vi "file list from temperatures file V3.vi"(6 "monotonic segments ON/OFF":bool=TRUE, 7 "action":T4(ring)=enum."update monotonic pieces", 9 "tfolder IN":T1={"tfolder path"=path "/snowfall/Users/arcadi/Desktop/Ultrasound/Experiment/YBCO_4/Round1/Sweep12/June_2011/062511/221.16400K_300_3100_001_062511.dat", "9folder path"=path "/snowfall/Users/arcadi/Desktop/Ultrasound/Experiment/YBCO_4/Round1/Sweep12/June_2011/062511/221.16400K_300_3100_001_062511.dat", "tfolder  -  file array"=[], "from index array"=[], "timestamp array"=[]}, 11 "tfolder file path  IN":path=path "/snowfall/Users/arcadi/Desktop/Ultrasound/Experiment/YBCO_4/Round1/Sweep12/June_2011/062511/221.16400K_300_3100_001_062511.dat") -> (0 "timestamp OUT":dbl[](array[numeric]), 1 "tfolder OUT":T1={"tfolder path"=path "/snowfall/Users/arcadi/Desktop/Ultrasound/Experiment/YBCO_4/Round1/Sweep12/June_2011/062511/221.16400K_300_3100_001_062511.dat", "9folder path"=path "/snowfall/Users/arcadi/Desktop/Ultrasound/Experiment/YBCO_4/Round1/Sweep12/June_2011/062511/221.16400K_300_3100_001_062511.dat", "tfolder  -  file array"=[], "from index array"=[], "timestamp array"=[]}, 2 "sweep path array OUT":T3[](array[typedef]), 3 "temperature OUT":dbl[](array[numeric]), 5 "OK":bool)   [LabVIEW 2010]
uses:
  sweep file name.ctl
  tfolder -- monotonic segment.ctl
  tfolder.ctl
panel:
  in  "tfolder - monotonic segment":T2
  in  "sweep file name":T3={"temperature"=0.0, "temperature str"="", "file path"=path "/snowfall/Users/arcadi/Desktop/Ultrasound/Experiment/YBCO_4/Round1/Sweep12/June_2011/062511/221.16400K_300_3100_001_062511.dat", "last mod"=timestamp(0 s since 1904-01-01), "file name str"="", "mod time(min)"=0.0, "file format"=enum.""}
  in  "file path OK":bool=TRUE
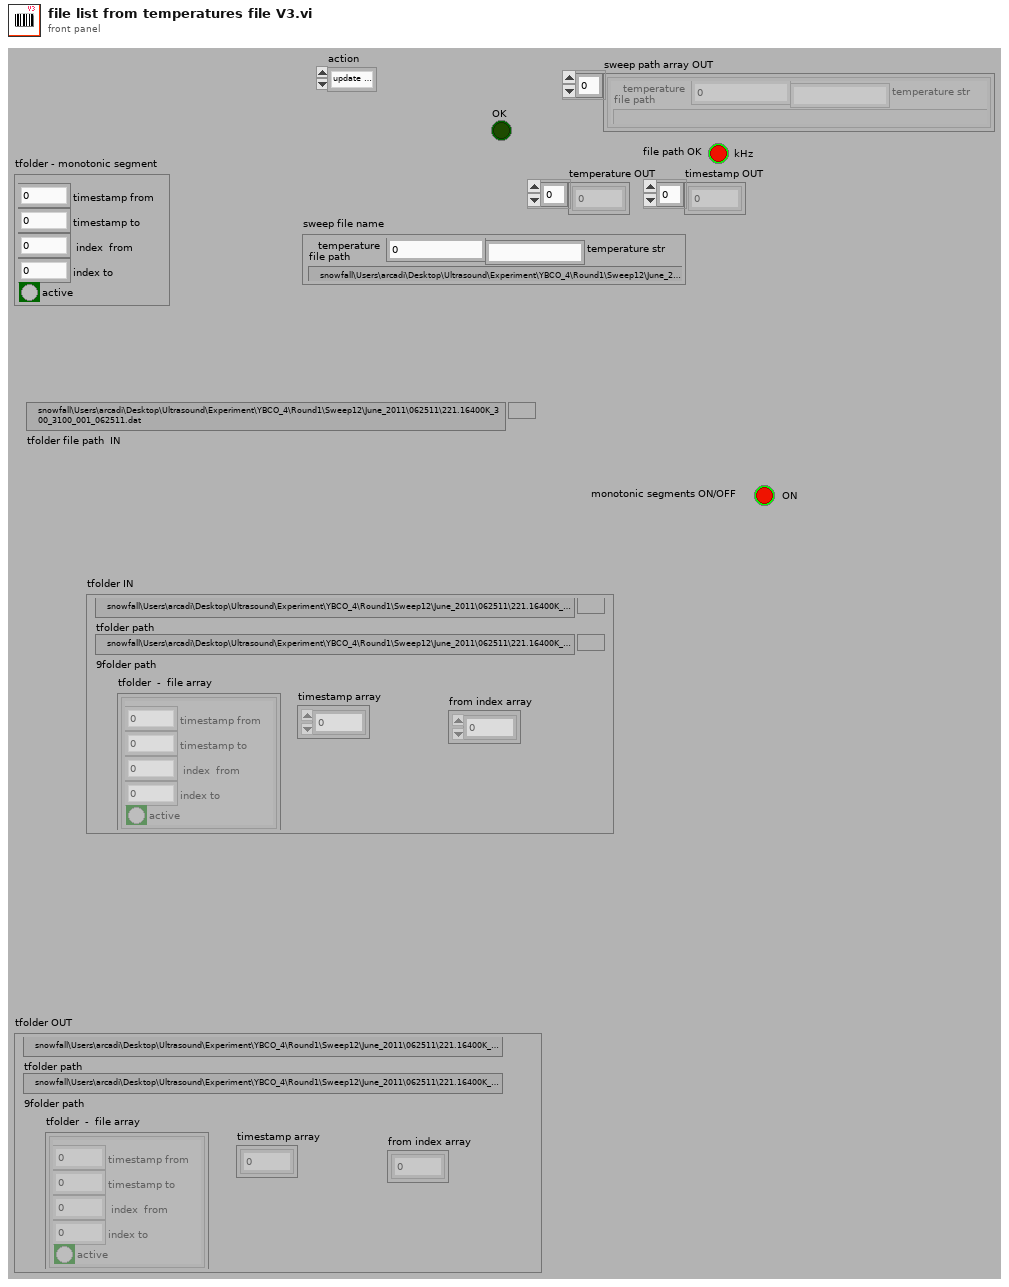
[diagram p1: front panel]
types:
  T1 = typedef "tfolder.ctl" = cluster{"tfolder path":path, "9folder path":path, "tfolder  -  file array":T2[], "from index array":i32[], "timestamp array":dbl[]}
  T2 = typedef "tfolder -- monotonic segment.ctl" = cluster{"timestamp from":dbl, "timestamp to":dbl, " index  from":i32, "index to":i32, "active":bool}
  T3 = typedef "sweep file name.ctl" = cluster{"temperature":dbl, "temperature str":string, "file path":path, "last mod":timestamp, "file name str":string, "mod time(min)":dbl, "file format":enum16{"", "ascii", "binary"}}
  T4 = enum16{"new", "update range", "update monotonic pieces", "init", "check", "reset", ""}
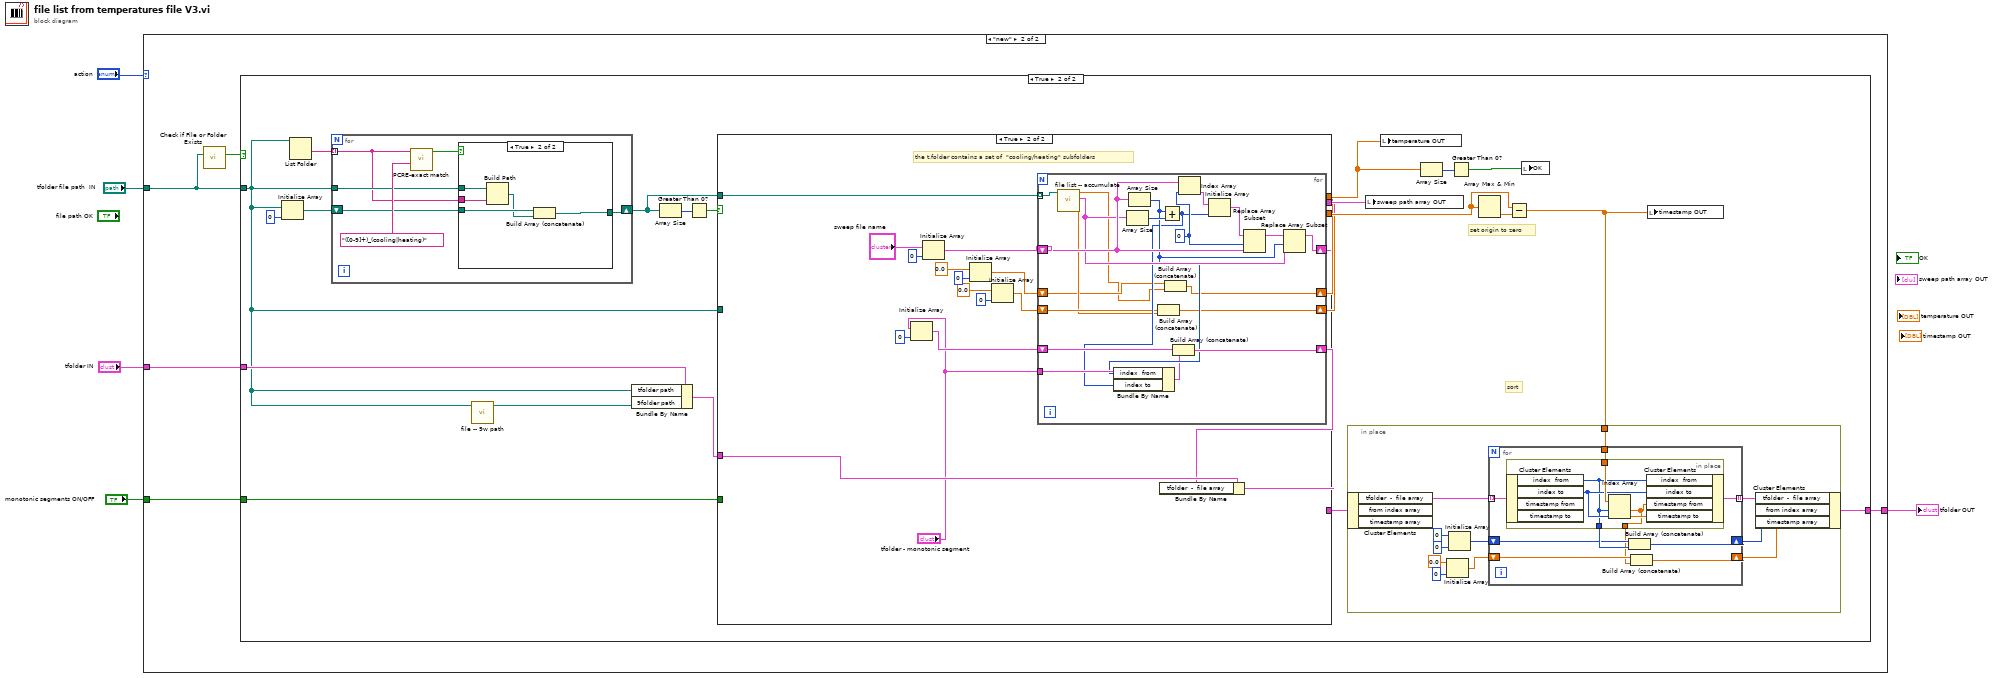
[diagram p0: block diagram]
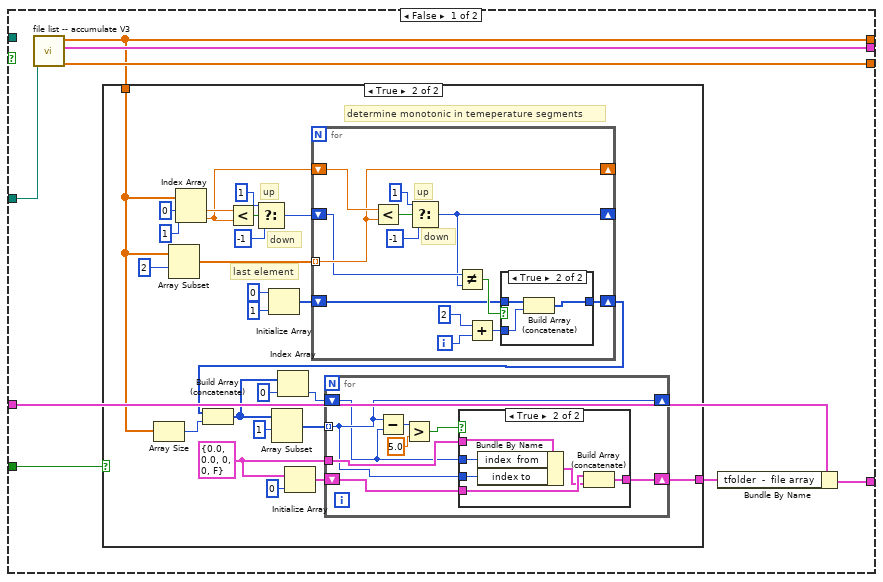
[diagram p4: hidden frame]
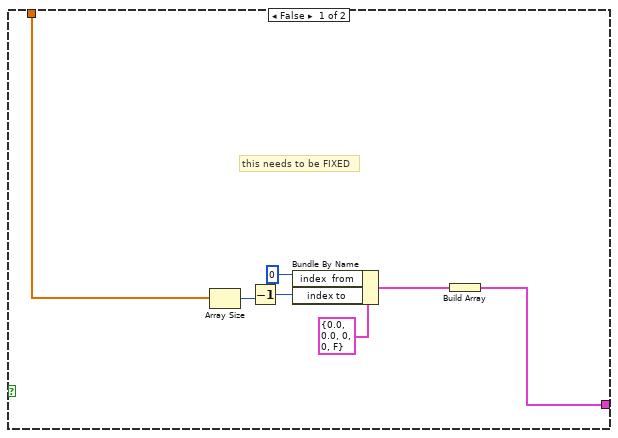
[diagram p5: hidden frame]
diagram:
  n1 = case shown="\"new\"" "action" {
    tunnel: "tfolder file path  IN" -> [_ w10]
    tunnel: "tfolder IN" -> [w6 w9]
    tunnel: [w6 w8] -> w2
    tunnel: "monotonic segments ON/OFF" -> [_ w7]
    frame "", Default {
    }
    frame "new" {
      n2 = call <vilib>:"Check if File or Folder Exists.vi"("path"=w10) -> ("file or folder exists?"=w11:bool)  [unwired: 8 in, 2 out]
      n3 = case shown="True" w11 {
        tunnel: w10 -> [_ w14]
        tunnel: w9 -> [w12 w26]
        tunnel: [w12 w20] -> w8
        tunnel: w7 -> [_ w18]
        frame False {
        }
        frame True {
          # "sort"
          # "set origin to zero"
          n4 = Initialize Array(w14, 0 ("dimension size")) -> (w30:path[])
          n5 = List Folder(path=w14) -> (folder names=w31:string[])  [unwired: 3 in, 3 out]
          n6 = for {
            tunnel: w31 -> [w172] mode=indexing
            shift-right: [w170] -> w27
            shift-left: w30 -> [w171]
            tunnel: w14 -> [w173]
            n7 = call "PCRE-exact match.vi"("regular expression"="([0-9]+)_(cooling|heating)", "input string"=w172) -> ("exact match"=w174:bool)  [unwired: 8 in, 1 out]
            n8 = case shown="True" w174 {
              tunnel: w173 -> [_ w181]
              tunnel: w172 -> [_ w180]
              tunnel: w171 -> [w176 w179]
              tunnel: [w176 w177] -> w170
              frame False {
              }
              frame True {
                n9 = Build Path(base path=w181, name or relative path=w180) -> (appended path=w178:path)
                n10 = Build Array (concatenate)(w179, w178) -> (w177:path[])
              }
            }
          }
          n11 = call "file -- 9w path.vi"("sweep folder"=w14) -> ("9w path"=w13:path)  [unwired: 10 in]
          n12 = Bundle By Name(cluster=w26, "tfolder path"=w14, "9folder path"=w13) -> (w24:T1)
          n13 = Array Size(array=w27) -> (size(s)=w29:i32)
          n14 = Greater Than 0?(x=w29) -> (x > 0?=w28:bool)
          n15 = case shown="True" w28 {
            tunnel: w27 -> [_ w148]
            tunnel: [w60 w147] -> w22
            tunnel: [w59 w146] -> w16
            tunnel: [w65 w145] -> w25
            tunnel: w24 -> [w63 w142]
            tunnel: [w62 w141] -> w21
            tunnel: w14 -> [w64 _]
            tunnel: w18 -> [w58 _]
            frame False {
              n16 = call "file list -- accumulate V3.vi"("file path"=w64) -> ("timestamp"=w60:dbl[], "sweep file name array"=w65:T3[], "temperatures"=w59:dbl[])  [unwired: 8 in]
              n17 = case shown="True" w58 {
                tunnel: [w66 w93] -> w61
                tunnel: w59 -> [w71 w73]
                frame False {
                  # "this needs to be FIXED"
                  n18 = Array Size(array=w71) -> (size(s)=w70:i32)
                  n19 = Decrement(x=w70) -> (x-1=w68:i32)
                  n20 = Bundle By Name(cluster=T2 {"timestamp from"=0.0, "timestamp to"=0.0, " index  from"=0, "index to"=0, "active"=FALSE} ("monotonic segment"), "index  from"=0, "index to"=w68) -> (w72:T2)
                  n21 = Build Array(w72) -> (w66:T2[])
                }
                frame True {
                  w94 = T2 {"timestamp from"=0.0, "timestamp to"=0.0, " index  from"=0, "index to"=0, "active"=FALSE} ("monotonic segment")
                  # "determine monotonic in temeperature segments"
                  # "last element"
                  # "down"
                  # "up"
                  n22 = Array Size(array=w73) -> (size(s)=w75:i32)
                  n23 = Array Subset(array=w73, index=2 ("dimension size")) -> (w87:dbl[])  [unwired: 1 in]
                  n24 = Index Array(array=w73, index #1=0 ("dimension size"), index #2=1 ("dimension size")) -> (element #1=w86:dbl, element #2=w85:dbl)
                  n25 = Less?(x=w86, y=w85) -> (x < y?=w77:bool)
                  n26 = Select(t=1 ("dimension size"), s=w77, f=-1 ("dimension size")) -> (s? t:f=w82:i32)
                  n27 = Initialize Array(0 ("dimension size"), 1 ("dimension size")) -> (w92:i32[])
                  n28 = Initialize Array(w94, 0 ("dimension size")) -> (w95:T2[])
                  n29 = for {
                    shift-right: [w98] -> w76
                    shift-left: w92 -> [w100]
                    shift-right: [w106] -> _
                    shift-left: w85 -> [w107]
                    tunnel: w87 -> [w106] mode=indexing
                    shift-right: [w102] -> _
                    shift-left: w82 -> [w103]
                    i -> [w105]
                    # "down"
                    # "up"
                    n30 = Less?(x=w107, y=w106) -> (x < y?=w110:bool)
                    n31 = Select(t=1 ("dimension size"), s=w110, f=-1 ("dimension size")) -> (s? t:f=w102:i32)
                    n32 = Not Equal?(x=w103, y=w102) -> (x != y?=w101:bool)
                    n33 = Add(x=2, y=w105) -> (x+y=w99:i32)
                    n34 = case shown="True" w101 {
                      tunnel: w100 -> [w111 w114]
                      tunnel: w99 -> [_ w113]
                      tunnel: [w111 w112] -> w98
                      frame False {
                      }
                      frame True {
                        n35 = Build Array (concatenate)(w114, w113) -> (w112:i32[])
                      }
                    }
                  }
                  n36 = Build Array (concatenate)(w76, w75) -> (w74:i32[])
                  n37 = Array Subset(array=w74, index=1 ("dimension size")) -> (w78:i32[])  [unwired: 1 in]
                  n38 = Index Array(array=w74, index=0 ("dimension size")) -> (element=w80:i32)
                  n39 = for {
                    shift-right: [w121] -> w93
                    shift-left: w95 -> [w122]
                    tunnel: w94 -> [w120]
                    shift-right: [w117] -> _
                    shift-left: w80 -> [w116]
                    tunnel: w78 -> [w117] mode=indexing
                    n40 = Subtract(x=w117, y=w116) -> (x-y=w119:i32)
                    n41 = Greater?(x=w119, y=5.0) -> (0:w115:bool)
                    n42 = case shown="True" w115 {
                      tunnel: w122 -> [w123 w129]
                      tunnel: [w123 w128] -> w121
                      tunnel: w120 -> [_ w126]
                      tunnel: w117 -> [_ w125]
                      tunnel: w116 -> [_ w124]
                      frame False {
                      }
                      frame True {
                        n43 = Bundle By Name(cluster=w126, "index  from"=w124, "index to"=w125) -> (w127:T2)
                        n44 = Build Array (concatenate)(w129, w127) -> (w128:T2[])
                      }
                    }
                  }
                }
              }
              n45 = Bundle By Name(cluster=w63, "tfolder  -  file array"=w61) -> (w62:T1)
            }
            frame True {
              # "the t.folder contains a set of  \"cooling/heating\" subfolders"
              n46 = Initialize Array("tfolder - monotonic segment", 0 ("dimension size")) -> (w143:T2[])
              n47 = Initialize Array("sweep file name", 0 ("dimension size")) -> (w134:T3[])
              n48 = Initialize Array(0.0 ("dimension size"), 0 ("dimension size")) -> (w133:dbl[])
              n49 = Initialize Array(0.0 ("dimension size"), 0 ("dimension size")) -> (w132:dbl[])
              n50 = for {
                tunnel: w148 -> [w169] mode=indexing
                shift-right: [w161] -> w145
                shift-left: w134 -> [w163]
                shift-right: [w149] -> w146
                shift-left: w133 -> [w151]
                shift-right: [w152] -> w147
                shift-left: w132 -> [w154]
                shift-right: [w159] -> w130
                shift-left: w143 -> [w160]
                tunnel: "tfolder - monotonic segment" -> [w158]
                w165 = 0 ("dimension size")
                n51 = call "file list -- accumulate.vi"("file path"=w169) -> ("timestamp"=w153:dbl[], "sweep file name array"=w162:T3[], "temperatures"=w150:dbl[])  [unwired: 8 in]
                n52 = Array Size(array=w162) -> (size(s)=w168:i32)
                n53 = Array Size(array=w163) -> (size(s)=w157:i32)
                n54 = Build Array (concatenate)(w154, w153) -> (w152:dbl[])
                n55 = Add(x=w157, y=w168) -> (x+y=w156:i32)
                n56 = Bundle By Name(cluster=w158, "index  from"=w157, "index to"=w156) -> (w155:T2)
                n57 = Build Array (concatenate)(w151, w150) -> (w149:dbl[])
                n58 = Build Array (concatenate)(w160, w155) -> (w159:T2[])
                n59 = Index Array(array=w163, index=w165) -> (element=w164:T3)
                n60 = Initialize Array(w164, w156) -> (w167:T3[])
                n61 = Replace Array Subset(array=w167, new element=w163, index=w165) -> (w166:T3[])
                n62 = Replace Array Subset(array=w166, new element=w162, index=w157) -> (w161:T3[])
              }
              n63 = Bundle By Name(cluster=w142, "tfolder  -  file array"=w130) -> (w141:T1)
            }
          }
          n64 = local write "sweep path array OUT"(w25) -> ()
          n65 = local write "temperature OUT"(w16) -> ()
          n66 = Array Size(array=w16) -> (size(s)=w17:i32)
          n67 = Greater Than 0?(x=w17) -> (x > 0?=w15:bool)
          n68 = Array Max & Min(array=w22) -> (min value=w23:dbl)  [unwired: 3 out]
          n69 = Subtract(x=w22, y=w23) -> (x-y=w19:dbl[])
          n70 = in-place {
            in-place-border: w19 -> [w42]
            n71 = in-place-cluster #1(w21) -> ("tfolder  -  file array"=w43:T2[])  [unwired: 2 out]
            n72 = Initialize Array(0.0 ("dimension size"), 0 ("dimension size")) -> (w36:dbl[])
            n73 = Initialize Array(0 ("dimension size"), 0 ("dimension size")) -> (w35:i32[])
            n74 = for {
              tunnel: w43 -> [w52] mode=indexing
              tunnel: w42 -> [w51]
              tunnel: [w50] -> w41 mode=indexing
              shift-right: [w45] -> w33
              shift-left: w35 -> [w47]
              shift-right: [w46] -> w34
              shift-left: w36 -> [w49]
              n75 = in-place {
                in-place-border: w51 -> [w57]
                in-place-border: [w54] -> w48
                in-place-border: [w53] -> w44
                n76 = in-place-cluster #2(w52) -> ("index  from"=w54:i32, "index to"=w55:i32)  [unwired: 2 out]
                n77 = Index Array(array=w57, index #1=w54, index #2=w55) -> (element #1=w53:dbl, element #2=w56:dbl)
                n78 = in-place-cluster #2("index  from"=w54, "index to"=w55, "timestamp from"=w53, "timestamp to"=w56) -> (w50:T2)
              }
              n79 = Build Array (concatenate)(w47, w48) -> (w45:i32[])
              n80 = Build Array (concatenate)(w49, w44) -> (w46:dbl[])
            }
            n81 = in-place-cluster #1("tfolder  -  file array"=w41, "from index array"=w33, "timestamp array"=w34) -> (w20:T1)
          }
          n82 = local write "OK"(w15) -> ()
          n83 = local write "timestamp OUT"(w19) -> ()
        }
      }
    }
  }
  "tfolder OUT" <- w2
